vi "Initialize.vi"(8 "error in":errorcluster, 10 "shared resources":refnum<class "Shared Resources.lvclass">, 11 "Rx execution unit in":refnum<class "Rx Execution Unit.lvclass">) -> (0 "error out":errorcluster, 3 "Rx execution unit out":refnum<class "Rx Execution Unit.lvclass">)   [LabVIEW 2020, in "AIM ARINC 429 Engine.lvlib" / "Implementation.lvlib" / "Rx Execution Unit.lvclass"]
uses:
  Rx Execution Unit.lvclass
  C:/Git/niveristand-aim-arinc429-custom-device/Source/Custom Device Support/Engine/Implementation/Execution Unit/Execution Unit.lvclass
  Interfaces/Shared Resources/Shared Resources.lvclass
  Shared Resources/Shared Resources.lvclass
  Shared Resources/Shared Resources.lvclass/Shared Resources.ctl
  Execution Unit/Execution Unit.lvclass/Execution Unit.ctl
  Rx Execution Unit.lvclass/Rx Execution Unit.ctl
  Custom Device/Custom Device.lvlib
  Execution Unit/Execution Unit.lvclass
  Hardware API/AIM ARINC 429 Hardware API.lvlib
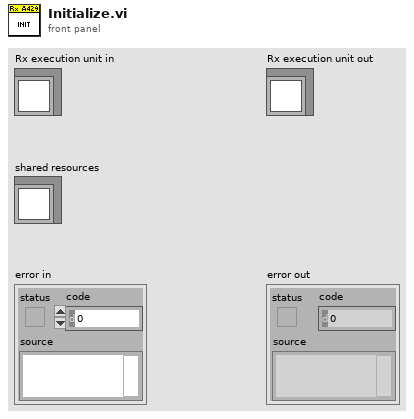
[diagram p1: front panel]
types:
  T1 = typedef "AIM ARINC 429 Engine.lvlib/Custom Device.lvlib/Hardware Handles.ctl" = cluster{"module":u8}
  T2 = typedef "RT Hardware Channel Settings.ctl" = cluster{"channel #":u16, "channel handle":u64, "labels settings for RT":T3[]}
  T3 = typedef "RT Label Settings.ctl" = cluster{"Name":string, "xmlName":string, "label":T4, "transfer period":u32, "SDI_Enabled":bool, "SDI":u8, "parameter driver data":T5, "transfer type":T9, "has timestamp?":bool, "Label Disable/Trigger Channel Reference":T8, "Message Handle":u64, "Initialized?":bool, "Word Initial Raw Value":u32, "Label Timestamp Channel Data Reference":T10, "disabled":bool}
  T4 = typedef "Label.ctl" = u8
  T5 = typedef "RT Parameters.ctl" = cluster{"parameter definitions":T6[], "Tx parameter refs":T8[]}
  T6 = typedef "Parameter Definition.ctl" = cluster{"start index":i32, "size":i32, "encoding":T7, "signed":bool, "scale multiplier":dbl, "scale offset":dbl}
  T7 = typedef "Encoding and Decoding.lvlib/Encoding.ctl" = enum16{"BNR", "BCD", "Discrete"}
  T8 = typedef "Custom Device API.lvlib/Custom Device Item Ref.ctl" = u64
  T9 = typedef "Transfer Type.ctl" = enum16{"Scheduled", "Acyclic", "Block", "Strobe"}
  T10 = typedef "Custom Device API.lvlib/Data Reference.ctl" = i32
  T11 = typedef "Map of Identifiers to Indexes.ctl" = map{cluster{"Port":u8, "Label":u8, "SDI":u8}, cluster{"channel index":i32, "label index":i32, "start index":i32, "parameters":i32, "timestamp index":i32}}
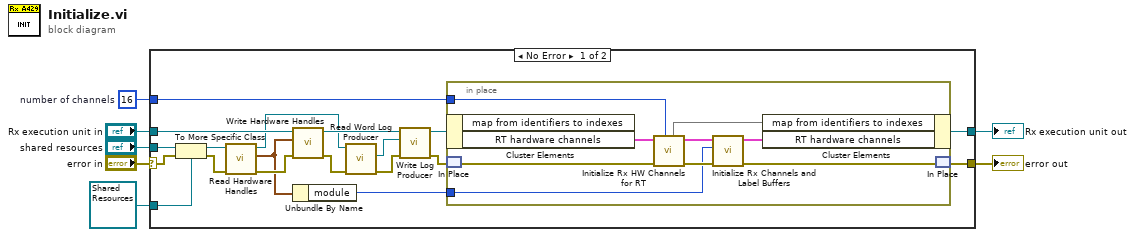
[diagram p0: block diagram]
diagram:
  w5 = 16  # number of channels
  n1 = case shown="No Error" "error in" {
    selector: "error in" -> [w16 w36]
    tunnel: "Rx execution unit in" -> [w23 w35]
    tunnel: [w26 w35] -> w6
    tunnel: w5 -> [w25 _]
    tunnel: [w20 w36] -> w4
    tunnel: "shared resources" -> [w18 _]
    tunnel: refnum<class "Shared Resources.lvclass"> refnum ("Ballard ARINC-429 shared resources in") -> [w19 _]
    frame No Error {
      n2 = To More Specific Class(target class=w19, reference=w18, error in=w16) -> (specific class reference=w17:refnum<class "Shared Resources.lvclass">, error out=w15:errorcluster)
      n3 = call "Read Hardware Handles.vi"("error in"=w15, "AIM ARINC-429 shared resources in"=w17) -> ("error out"=w22:errorcluster, "hardware handles"=w10:T1, "AIM ARINC-429 shared resources out"=w8:refnum<class "Shared Resources.lvclass">)  [unwired: 7 in]
      n4 = call "Write Hardware Handles.vi"("error in"=w22, "hardware handles"=w10, "AIM ARINC-429 execution unit in"=w23) -> ("error out"=w21:errorcluster, "AIM ARINC-429 execution unit out"=w24:refnum<class "Rx Execution Unit.lvclass">)  [unwired: 7 in]
      n5 = Unbundle By Name(w10) -> ("module"=w9:u8)
      n6 = call-dynamic "Read Word Log Producer.vi"("error in"=w21, "shared resources in"=w8) -> ("error out"=w13:errorcluster, "word log producer"=w11:refnum<class "Log Producer.lvclass">)  [unwired: 7 in, 1 out]
      n7 = call-dynamic "Write Log Producer.vi"("error in (no error)"=w13, "Log Producer"=w11, "Rx Execution Unit in"=w24) -> ("error out"=w12:errorcluster, "Rx Execution Unit out"=w14:refnum<class "Rx Execution Unit.lvclass">)  [unwired: 7 in]
      n8 = in-place {
        in-place-border: w25 -> [w34]
        in-place-border: w9 -> [w27]
        n9 = in-place-cluster #1(w14) -> ("RT hardware channels"=w33:T2[])  [unwired: 1 out]
        n10 = in-place-match #2(w12) -> (w29:errorcluster)
        n11 = call "Initialize Rx HW Channels for RT.vi"("number of channels"=w34, "Rx Channels In"=w33) -> ("Rx Channels Out"=w31:T2[], "map from identifiers to indexes"=w32:T11)  [unwired: 6 in]
        n12 = call "Initialize Rx Channels and Label Buffers.vi"("error in"=w29, "module handle"=w27, "Rx Channels Out in"=w31) -> ("error out"=w28:errorcluster, "Rx Channels Out out"=w30:T2[])  [unwired: 7 in]
        n13 = in-place-cluster #1("map from identifiers to indexes"=w32, "RT hardware channels"=w30) -> (w26:refnum<class "Rx Execution Unit.lvclass">)
        n14 = in-place-match #2(w28) -> (w20:errorcluster)
      }
    }
    frame Error {
    }
  }
  "error out" <- w4
  "Rx execution unit out" <- w6
